vi "Instrument AutoScale (LTE).vi"(4 "Perform AutoScale (T)":bool, 8 "error in":errorcluster {"code" format="%.0x"}, 10 "AUTOSCALE ON/OFF":string(combo)="ON", 11 "Session In":refnum<visa-resource-name>="GPIB0::18::INSTR") -> (0 "error out":errorcluster {"code" format="%.0x"}, 3 "Session Out":refnum<visa-resource-name>, 6 "ON/OFF":string)   [LabVIEW 2018]
doc: "Launches the Instrument I/O Assistant, which you can use to communicate with message-based instruments and graphically parse the response. For example you can communicate with an instrument that uses a serial, Ethernet, or GPIB interface."
panel:
  in  "RO(T)":bool
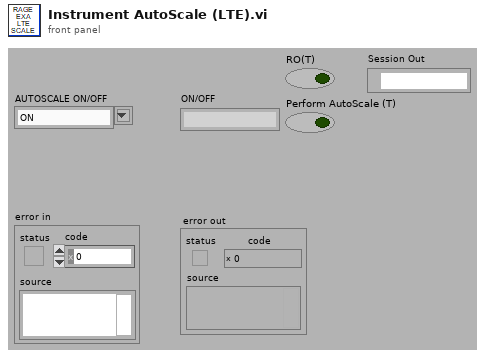
[diagram p1: front panel]
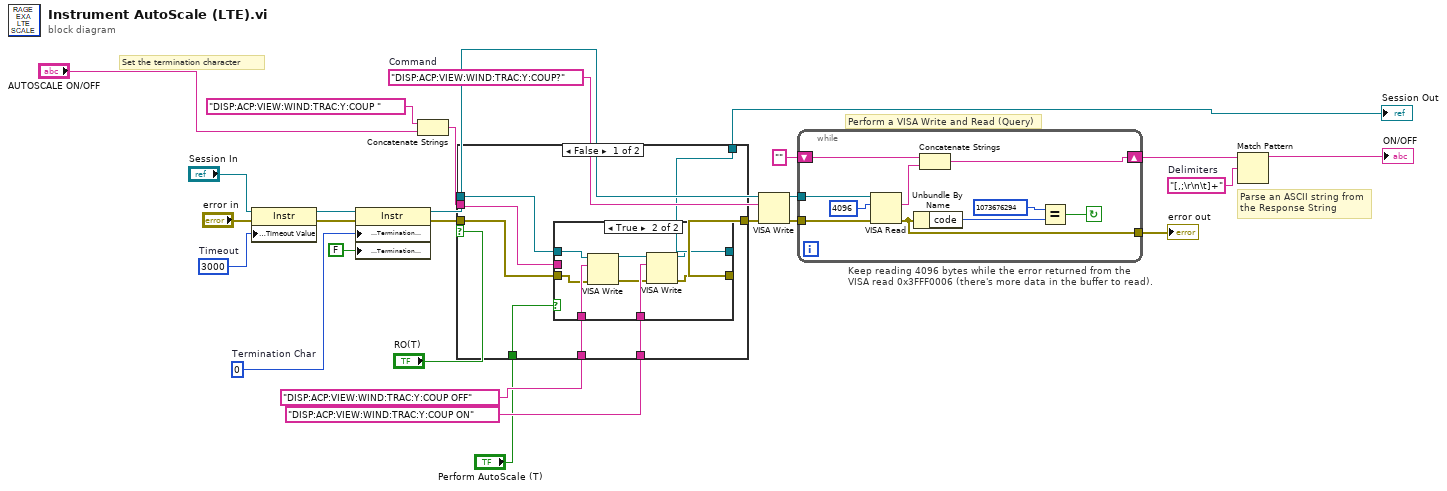
[diagram p0: block diagram]
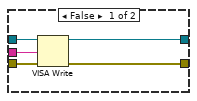
[diagram p2: hidden frame]
diagram:
  w8 = "[,;\r\n\t]+"  # Delimiters
  w10 = "DISP:ACP:VIEW:WIND:TRAC:Y:COUP?"  # Command
  w21 = u8 0  # Termination Char
  w25 = u32 3000  # Timeout
  # "Parse an ASCII string from the Response String"
  # "Perform a VISA Write and Read (Query)"
  # "Keep reading 4096 bytes while the error returned from the\nVISA read 0x3FFF0006 (there's more data in the buffer to read)."
  # "Set the termination character"
  n1 = property class="Instr"(reference="Session In", error in="error in", "General Settings:Timeout Value"=w25) -> (reference out=w20:refnum<visa-resource-name>, error out=w23:errorcluster)
  n2 = property class="Instr"(reference=w20, error in=w23, "Message Based Settings:Termination Character"=w21, "Message Based Settings:Termination Character Enable"=FALSE ("enable")) -> (reference out=w6:refnum<visa-resource-name>, error out=w22:errorcluster)
  n3 = Concatenate Strings("DISP:ACP:VIEW:WIND:TRAC:Y:COUP " ("staticText"), "AUTOSCALE ON/OFF") -> (w15:string)
  n4 = case shown="False" "RO(T)" {
    tunnel: w22 -> [w30 w49]
    tunnel: [w34 w49] -> w16
    tunnel: w15 -> [w33 _]
    tunnel: w6 -> [w32 w48]
    tunnel: [w31 w48] -> w5
    tunnel: "DISP:ACP:VIEW:WIND:TRAC:Y:COUP OFF" ("staticText") -> [w29 _]
    tunnel: "DISP:ACP:VIEW:WIND:TRAC:Y:COUP ON" ("staticText") -> [w28 _]
    tunnel: "Perform AutoScale (T)" -> [w27 _]
    frame False {
      n5 = case shown="True" w27 {
        tunnel: [w39 w41] -> w34
        tunnel: w33 -> [w38 _]
        tunnel: w32 -> [w37 w46]
        tunnel: [w36 w40] -> w31
        tunnel: w30 -> [w35 w45]
        tunnel: w29 -> [_ w47]
        tunnel: w28 -> [_ w44]
        frame False {
          n6 = VISA Write(VISA resource name=w37, write buffer=w38, error in (no error)=w35) -> (VISA resource name out=w36:refnum<visa-resource-name>, error out=w39:errorcluster)  [unwired: 1 out]
        }
        frame True {
          n7 = VISA Write(VISA resource name=w46, write buffer=w47, error in (no error)=w45) -> (VISA resource name out=w43:refnum<visa-resource-name>, error out=w42:errorcluster)  [unwired: 1 out]
          n8 = VISA Write(VISA resource name=w43, write buffer=w44, error in (no error)=w42) -> (VISA resource name out=w40:refnum<visa-resource-name>, error out=w41:errorcluster)  [unwired: 1 out]
        }
      }
    }
    frame True {
    }
  }
  "Session Out" <- w5
  n9 = VISA Write(VISA resource name=w6, write buffer=w10, error in (no error)=w16) -> (VISA resource name out=w14:refnum<visa-resource-name>, error out=w13:errorcluster)  [unwired: 1 out]
  n10 = while {
    tunnel: w14 -> [w56]
    shift-right: [w50] -> w7
    shift-left: "" -> [w55]
    tunnel: w13 -> [w53]
    tunnel: [w52] -> w12
    stop <- w51 continue-if-true
    n11 = VISA Read(VISA resource name=w56, byte count=u32 4096 ("byte count (0)"), error in (no error)=w53) -> (read buffer=w54:string, error out=w52:errorcluster)  [unwired: 2 out]
    n12 = Unbundle By Name(w52) -> ("code"=w58:i32)
    n13 = Concatenate Strings(w55, w54) -> (w50:string)
    n14 = Equal?(x=1073676294, y=w58) -> (x = y?=w51:bool)
  }
  "error out" <- w12
  n15 = Match Pattern(string=w7, regular expression=w8) -> (before substring=→"ON/OFF":string)  [unwired: 4 out]
